vi "practica robot1.vi"() -> ()   [LabVIEW 2017]
panel:
  out "Array 4":dbl[](array[numeric])
  out "Array 3":dbl[](array[numeric])
  out "Array 2":dbl[](array[numeric])
  out "Array":dbl[](array[numeric])
  in  "S2":i32
  in  "S1":i32
  in  "stop":bool
  in  "S2":dbl(knob) scale=-175.0..175.0
  in  "S1":dbl(knob) scale=0.0..360.0
  out "XY Graph":cluster{"Y":dbl[], "Y":dbl[]}[](graph)
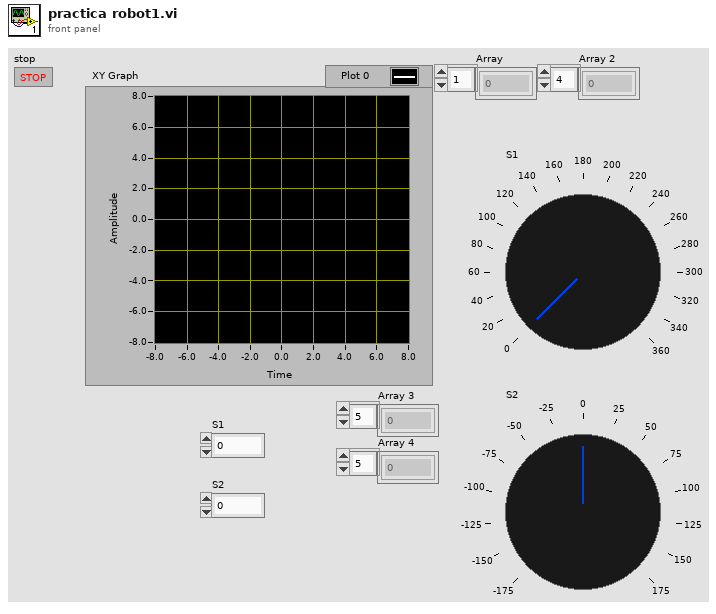
[diagram p1: front panel]
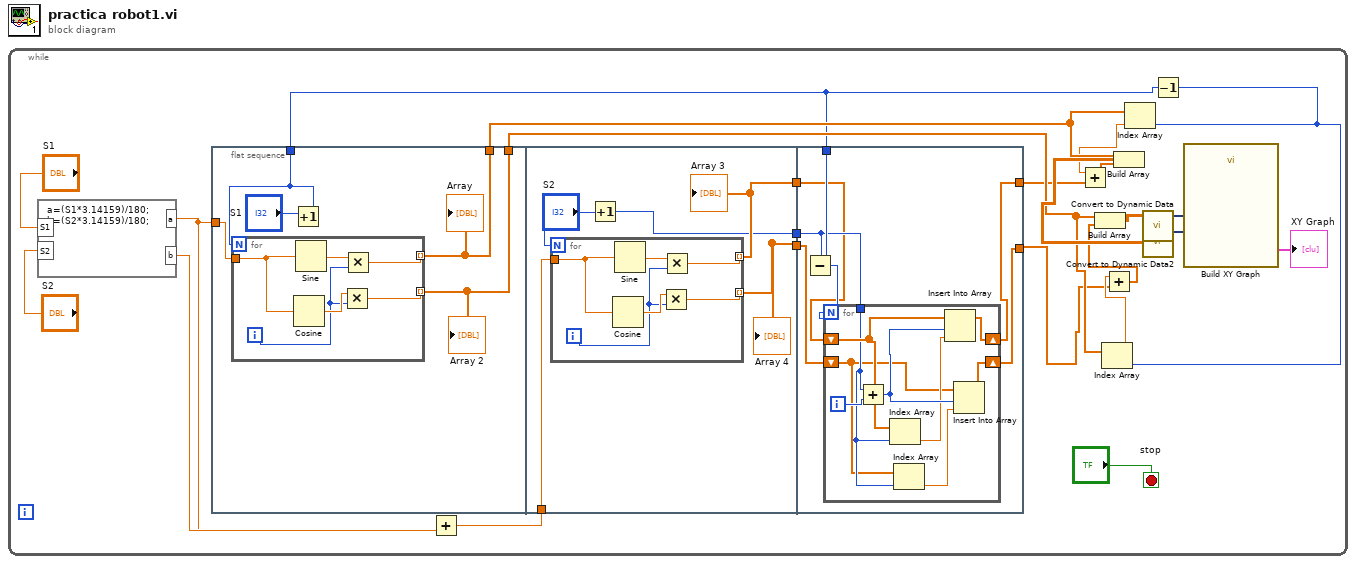
[diagram p0: block diagram]
diagram:
  n1 = while {
    stop <- "stop" stop-if-true
    n2 = formula code="a=(S1*3.14159)/180;\nb=(S2*3.14159)/180;"("S1"="S1", "S2"="S2") -> ("b"=w12:dbl, "a"=w11:dbl)
    n3 = flat-sequence {
      tunnel: w11 -> [w29]
      tunnel: [w25] -> w2
      tunnel: [w27] -> w10
      tunnel: [w26] -> w9
      tunnel: w8 -> [w39]
      tunnel: [w38] -> w4
      tunnel: [w37] -> w3
      tunnel: [w36] -> w1
      tunnel: [w48] -> w6
      tunnel: [w47] -> w7
      tunnel: w4 -> [w49]
      tunnel: w3 -> [w50]
      tunnel: w2 -> [w53]
      tunnel: w1 -> [w51]
      frame #0 {
        n4 = Increment(x="S1") -> (x+1=w25:i32)
        n5 = for {
          N: w25 -> [_]
          tunnel: w29 -> [w31]
          tunnel: [w33] -> w27 mode=indexing
          tunnel: [w32] -> w26 mode=indexing
          i -> [w30]
          n6 = Cosine(x=w31) -> (cos(x)=w35:dbl)
          n7 = Sine(x=w31) -> (sin(x)=w34:dbl)
          n8 = Multiply(x=w35, y=w30) -> (x*y=w32:dbl)
          n9 = Multiply(x=w34, y=w30) -> (x*y=w33:dbl)
        }
        "Array" <- w27
        "Array 2" <- w26
      }
      frame #1 {
        n10 = Increment(x="S2") -> (x+1=w36:i32)
        n11 = for {
          N: w36 -> [_]
          tunnel: w39 -> [w42]
          tunnel: [w44] -> w37 mode=indexing
          tunnel: [w43] -> w38 mode=indexing
          i -> [w41]
          n12 = Cosine(x=w42) -> (cos(x)=w46:dbl)
          n13 = Sine(x=w42) -> (sin(x)=w45:dbl)
          n14 = Multiply(x=w46, y=w41) -> (x*y=w43:dbl)
          n15 = Multiply(x=w45, y=w41) -> (x*y=w44:dbl)
        }
        "Array 3" <- w37
        "Array 4" <- w38
      }
      frame #2 {
        n16 = Subtract(x=w53, y=w51) -> (x-y=w52:i32)
        n17 = for {
          N: w52 -> [_]
          tunnel: w51 -> [w57]
          shift-right: [w58] -> w48
          shift-left: w50 -> [w60]
          shift-right: [w54] -> w47
          shift-left: w49 -> [w56]
          i -> [w62]
          n18 = Add(x=w57, y=w62) -> (x+y=w61:i32)
          n19 = Index Array(array=w60, index=w57) -> (element=w59:dbl)
          n20 = Index Array(array=w56, index=w57) -> (element=w55:dbl)
          n21 = Insert Into Array(array=w60, index=w61, new element=w59) -> (w58:dbl[])
          n22 = Insert Into Array(array=w56, index=w61, new element=w55) -> (w54:dbl[])
        }
      }
    }
    n23 = Add(x=w11, y=w12) -> (x+y=w8:dbl)
    n24 = Decrement(x=w2) -> (x-1=w13:i32)
    n25 = Index Array(array=w9, index=w13) -> (element=w14:dbl)
    n26 = Add(x=w14, y=w7) -> (x+y=w15:dbl[])
    n27 = Build Array(w9, w15) -> (w21:dbl[][])
    n28 = Index Array(array=w10, index=w13) -> (element=w5:dbl)
    n29 = Add(x=w5, y=w6) -> (x+y=w16:dbl[])
    n30 = Build Array(w10, w16) -> (w19:dbl[][])
    n31 = call "Convert to Dynamic Data"("2D Array"=w21) -> ("Dynamic Data Type"=w20:dynamicdata)  [unwired: 3 in]
    n32 = call "Convert to Dynamic Data2"("2D Array"=w19) -> ("Dynamic Data Type"=w18:dynamicdata)  [unwired: 3 in]
    n33 = call "Build XY Graph"("Y Input"=w18, "X Input"=w20) -> ("XY Graph"=→"XY Graph":cluster{"X":dbl[], "Y":dbl[]}[])  [unwired: 8 in, 1 out]
  }
